vi "Run.vi"(8 "error in (no error)":errorcluster, 11 "socket SUB in":refnum<class "socket SUB.lvclass">) -> (0 "error out":errorcluster, 3 "socket SUB out":refnum<class "socket SUB.lvclass">)   [LabVIEW 2018, in "socket SUB.lvclass"]
uses:
  socket SUB.lvclass
  Socket/Socket.lvclass
  State Machine/State Machine.lvclass
  RxTx/RxTx.lvclass
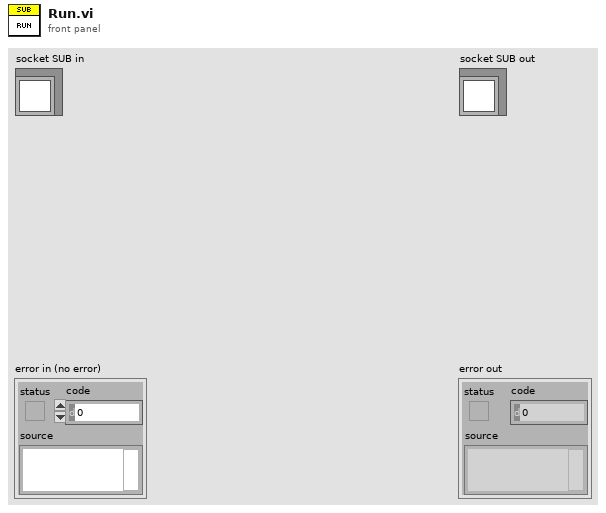
[diagram p1: front panel]
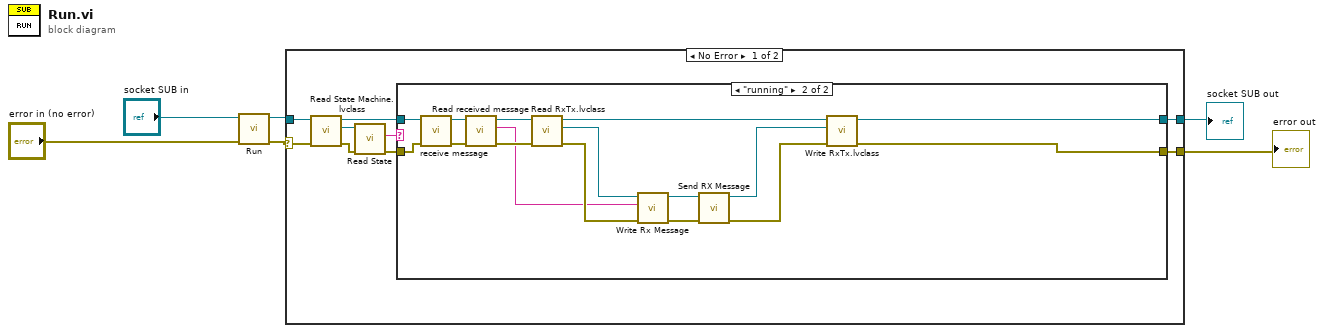
[diagram p0: block diagram]
diagram:
  n1 = call-parent "Run.vi"("error in (no error)"="error in (no error)", "Socket in"="socket SUB in") -> ("error out"=w3:errorcluster, "Socket out"=w4:refnum<class "socket SUB.lvclass">)  [unwired: 8 in]
  n2 = case shown="No Error" w3 {
    selector: w3 -> [w9 w33]
    tunnel: w4 -> [w10 w34]
    tunnel: [w13 w34] -> w2
    tunnel: [w14 w33] -> w1
    frame No Error {
      n3 = call-dynamic "Read State Machine.lvclass.vi"("error in (no error)"=w9, "Socket in"=w10) -> ("error out"=w8:errorcluster, "State Machine.lvclass"=w11:refnum<class "State Machine.lvclass">, "Socket out"=w7:refnum<class "socket SUB.lvclass">)  [unwired: 7 in]
      n4 = call-dynamic "Read State.vi"("error in (no error)"=w8, "State Machine in"=w11) -> ("error out"=w12:errorcluster, "State"=w15:string)  [unwired: 7 in, 1 out]
      n5 = case shown="\"running\"" w15 {
        tunnel: [w16 w19] -> w13
        tunnel: [w17 w18] -> w14
        tunnel: w12 -> [w17 w23]
        tunnel: w7 -> [w16 w24]
        frame Default {
        }
        frame "running" {
          n6 = call-dynamic "receive message.vi"("error in (no error)"=w23, "Socket in"=w24) -> ("error out"=w31:errorcluster, "Socket out"=w32:refnum<class "socket SUB.lvclass">)  [unwired: 8 in]
          n7 = call-dynamic "Read received message.vi"("error in (no error)"=w31, "Socket in"=w32) -> ("error out"=w29:errorcluster, "received message"=w28:string, "Socket out"=w25:refnum<class "socket SUB.lvclass">)  [unwired: 7 in]
          n8 = call-dynamic "Read RxTx.lvclass.vi"("Socket in"=w25) -> ("RxTx.lvclass"=w26:refnum<class "RxTx.lvclass">, "Socket out"=w21:refnum<class "socket SUB.lvclass">)  [unwired: 8 in, 1 out]
          n9 = call "Write Rx Message.vi"("error in (no error)"=w29, "Rx Message"=w28, "RxTx in"=w26) -> ("error out"=w27:errorcluster, "RxTx out"=w30:refnum<class "RxTx.lvclass">)  [unwired: 7 in]
          n10 = call "Send RX Message.vi"("error in (no error)"=w27, "RxTx in"=w30) -> ("error out"=w20:errorcluster, "RxTx out"=w22:refnum<class "RxTx.lvclass">)  [unwired: 8 in]
          n11 = call-dynamic "Write RxTx.lvclass.vi"("error in (no error)"=w20, "RxTx.lvclass"=w22, "Socket in"=w21) -> ("error out"=w18:errorcluster, "Socket out"=w19:refnum<class "socket SUB.lvclass">)  [unwired: 7 in]
        }
      }
    }
    frame Error {
    }
  }
  "error out" <- w1
  "socket SUB out" <- w2
